vi "main_switch.vi"() -> ()   [LabVIEW 2018]
uses:
  <instrlib>/Keithley 622x LV 2009/Configure/Source/Typedefs/KE622x -- Voltage Limit.ctl
  <instrlib>/Keithley 622x LV 2009/Configure/Output/Typedefs/KE6221 -- Output Response.ctl
  <instrlib>/Keithley 622x LV 2009/Utility/Typedefs/KE622x -- Instrument Type.ctl
  <instrlib>/Keithley 622x LV 2009/Typedefs/KE622x -- On Off Control.ctl
  <instrlib>/Keithley 622x LV 2009/Configure/Source/Typedefs/KE622x -- Current Range.ctl
  <instrlib>/Keithley 622x LV 2009/Configure/Source/Typedefs/KE622x -- Current Ranges.ctl
  <instrlib>/Keithley 622x LV 2009/Configure/Source/Typedefs/KE622x -- Current Level.ctl
  <vilib>/Utility/file.llb/Write Delimited Spreadsheet (string).vi
  <instrlib>/Keithley 622x LV 2009/Keithley 622x.lvlib
  <instrlib>/Keithley 2182/Keithley 2182.lvlib
panel:
  in  "VISA Switch":refnum<visa-resource-name>="GPIB::6"
  out "Close Channel List":string
  in  "Configurations":enum32{"Radio Selection 1", "Radio Selection 2"}(radio)
  out "Iteration number":i32
  out "Current  (A)":dbl
  out "Array Voltage  (V)":dbl
  in  "Voltage Resolution (8)":i32=8
  in  "Range Value (10)":dbl=10.0
  in  "Autorange (T: Enable)":bool=TRUE
  in  "Integration Rate (5)":dbl=5.0
  in  "Integration Rate Units (0: Line Cycles)":i32(ring) items=["Line Cycles", "Seconds"]
  in  "Buffer Count":i32=1
  in  "VISA resource voltage":refnum<visa-resource-name>
  out "Buffer":dbl[](array[numeric])
  out "Buffer Metadata":T1(array[cluster])
  in  "Measurement (0: Voltage Channel 1)":i32(ring) items=["Voltage Channel 1", "Voltage Channel 2"]
  in  "milliseconds to wait":u32=1000
  in  "Step Size":T2=0.001 min=-0.105 max=0.105 format="%.4p"
  in  "End":T2=0.001 min=-0.105 max=0.105 format="%.4p"
  in  "Start":T2=0.001 min=-0.105 max=0.105 format="%.4p"
  in  "Turn Off Output If Voltage Limit?":bool=TRUE
  out "Interlock Tripped?":bool
  out "Voltage Limit?":bool
  in  "Check For SCPI Errors? (T)":bool=TRUE
  in  "Current Range In":T3={"Auto Range?"=TRUE, "Man / Selected\nRange"=enum."2nA"}
  in  "Analog Filter State":T5
  in  "Output Response":T6=enum."Slow"
  in  "Voltage Limit (V)":T7=10.0 min=0.1 max=105.0 step=0.01 format="%.2p"
  out "error at Current off":errorcluster
  out "error at current On":errorcluster
  in  "VISA resource dc ac current source (16)":refnum<visa-resource-name>
  out "Configuration Error":errorcluster
  in  "array":dbl[](array[numeric])
  out "output array":dbl[](array[numeric])
  in  "Instrument Type 2":T8=enum."KE6221"
  # "( select : GPIB0::16::INSTR )"
  # "( select : GPIB0::25::INSTR )"
  # "( select : USB0::0x05E6::0x3706::04368238::INSTR )"
  # "Do Not Enter Buffer Size less than 2"
types:
  T1 = cluster{"Units":string, "Channel":i32, "Channel Type":string}[]
  T2 = typedef "Keithley 622x.lvlib/KE622x -- Current Level.ctl" = dbl
  T3 = typedef "Keithley 622x.lvlib/KE622x -- Current Range.ctl" = cluster{"Auto Range?":bool, "Man / Selected\nRange":T4}
  T4 = typedef "Keithley 622x.lvlib/KE622x -- Current Ranges.ctl" = enum16{"2nA", "20nA", "200nA", "2uA", "20uA", "200uA", "2mA", "20mA", "100mA"}
  T5 = typedef "Keithley 622x.lvlib/KE622x -- On Off Control.ctl" = enum16{"Off", "On"}
  T6 = typedef "Keithley 622x.lvlib/KE6221 -- Output Response.ctl" = enum16{"Fast", "Slow"}
  T7 = typedef "Keithley 622x.lvlib/KE622x -- Voltage Limit.ctl" = dbl
  T8 = typedef "Keithley 622x.lvlib/KE622x -- Instrument Type.ctl" = enum16{"KE6220", "KE6221"}
  T9 = enum16{"Close", "Close Exclusive", "Close Slot Exclusive", "Open", "Open All"}
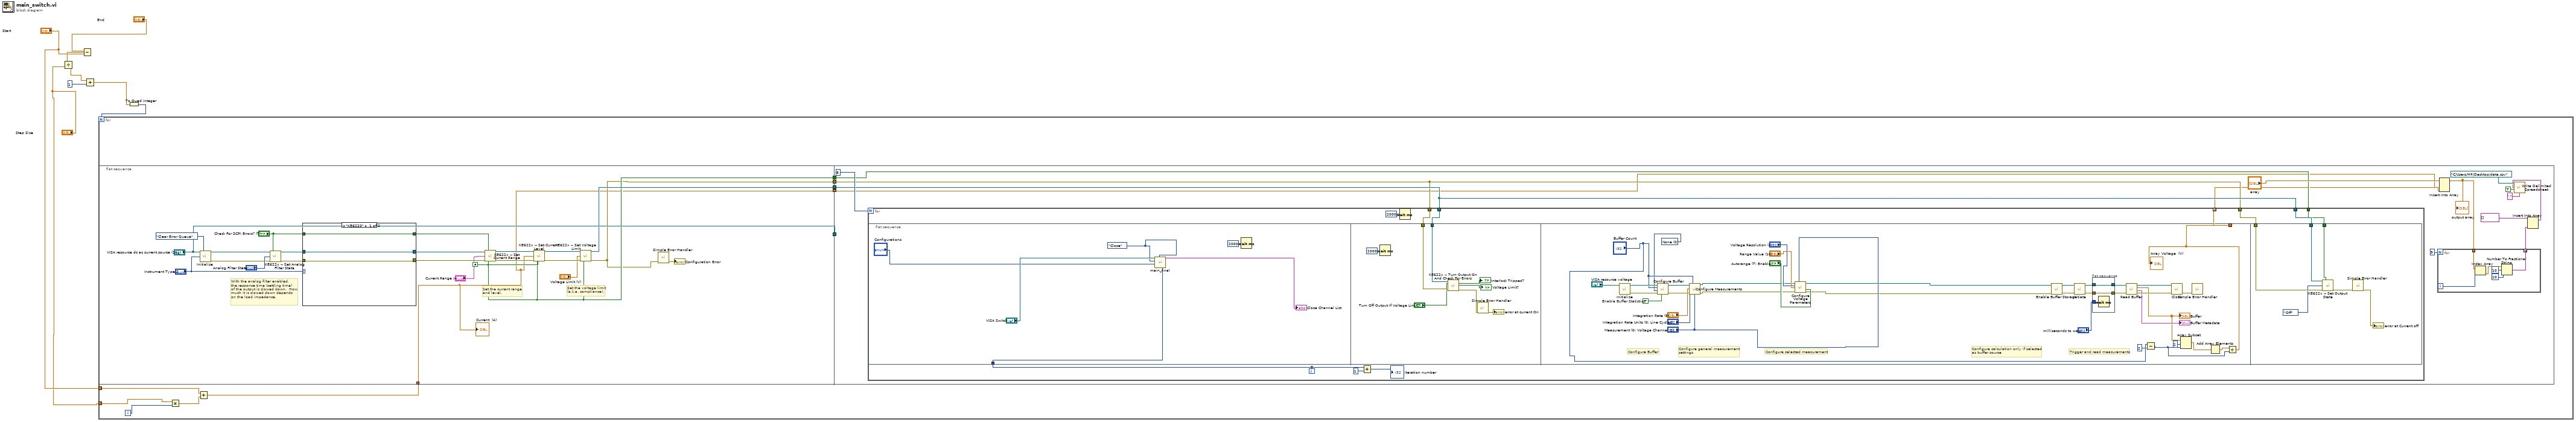
[diagram p0: block diagram]
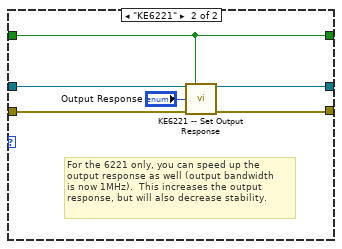
[diagram p2: hidden frame]
diagram:
  n1 = Subtract(x="End", y="Start") -> (x-y=w8:T2)
  n2 = Divide(x=w8, y="Step Size") -> (x/y=w4:T2)
  n3 = Add(x=w4, y=1) -> (x+y=w2:T2)
  n4 = To Quad Integer(1:w2) -> (0:w1:i64)
  n5 = for {
    N: w1 -> [_]
    tunnel: "Step Size" -> [w13]
    tunnel: "Start" -> [w12]
    i -> [w9]
    n6 = flat-sequence {
      tunnel: ["VISA resource dc ac current source (16)"] -> w18
      tunnel: [w22] -> w17
      tunnel: [w20] -> w16
      tunnel: [w21] -> w15
      tunnel: [w19] -> w14
      tunnel: w11 -> [w19]
      tunnel: w18 -> [_]
      tunnel: w17 -> [w63]
      tunnel: w16 -> [w62]
      tunnel: w15 -> [w61]
      tunnel: w14 -> [w51]
      frame #0 {
        w29 = FALSE ("Read Back Set Values? (T)")
        # "Set the voltage limit\n(a.k.a. compliance)."
        # "Set the current range\nand level."
        # "With the analog filter enabled,\nthe response time (settling time)\nof the output is slowed down.  How\nmuch it is slowed down depends\non the load impedance."
        n7 = call <instrlib>:"Initialize.vi"("VISA resource name"="VISA resource dc ac current source (16)", "Error Queue Option"=enum16{"Clear Error Queue", "Error Query"}."Clear Error Queue", "Instrument Type"="Instrument Type 2") -> ("VISA resource name out"=w39:refnum<visa-resource-name>, "error out"=w38:errorcluster)  [unwired: 11 in]
        n8 = call <instrlib>:"KE622x -- Set Analog Filter State.vi"("Resource In"=w39, "Check For SCPI Errors? (T)"="Check For SCPI Errors? (T)", "Analog Filter State"="Analog Filter State", "error in (no error)"=w38) -> ("Resource Out (dupl)"=w37:refnum<visa-resource-name>, "error out"=w35:errorcluster)  [unwired: 10 in]
        n9 = case shown="\"KE6220\"" "Instrument Type 2" {
          tunnel: w37 -> [w43 w50]
          tunnel: w35 -> [w42 w48]
          tunnel: [w43 w47] -> w32
          tunnel: "Check For SCPI Errors? (T)" -> [w44 w46]
          tunnel: [w44 w46] -> w21
          tunnel: [w42 w45] -> w33
          frame "KE6220" {
          }
          frame "KE6221" {
            # "For the 6221 only, you can speed up the\noutput response as well (output bandwidth\nis now 1MHz).  This increases the output\nresponse, but will also decrease stability."
            n10 = call <instrlib>:"KE6221 -- Set Output Response.vi"("Resource In"=w50, "Check For SCPI Errors? (T)"=w46, "KE6221 Output Response"="Output Response", "error in (no error)"=w48) -> ("Resource Out (dupl)"=w47:refnum<visa-resource-name>, "error out"=w45:errorcluster)  [unwired: 10 in]
          }
        }
        n11 = call <instrlib>:"KE622x -- Set Current Range.vi"("Resource In"=w32, "Check For SCPI Errors? (T)"=w21, "Current Range In"="Current Range In", "error in (no error)"=w33, "Read Back Set Values? (T)"=w29) -> ("Resource Out (dupl)"=w31:refnum<visa-resource-name>, "error out"=w30:errorcluster)  [unwired: 8 in, 1 out]
        n12 = call <instrlib>:"KE622x -- Set Current Level.vi"("Resource In"=w31, "Check For SCPI Errors? (T)"=w21, "Current Level (A) In"=w19, "error in (no error)"=w30, "Read Back Set Value? (T)"=w29) -> ("Resource Out (dupl)"=w28:refnum<visa-resource-name>, "error out"=w27:errorcluster)  [unwired: 8 in, 1 out]
        n13 = call <instrlib>:"KE622x -- Set Voltage Limit.vi"("Resource In"=w28, "Check For SCPI Errors? (T)"=w21, "Voltage Limit (V)"="Voltage Limit (V)", "error in (no error)"=w27) -> ("Resource Out (dupl)"=w22:refnum<visa-resource-name>, "error out"=w20:errorcluster)  [unwired: 10 in]
        n14 = call <vilib>:"Simple Error Handler.vi"("error in (no error)"=w20) -> ("error out"=→"Configuration Error":errorcluster)  [unwired: 4 in, 4 out]
        "Current  (A)" <- w19
      }
      frame #1 {
        n15 = for {
          N: 8 -> [_]
          tunnel: [w80] -> w52 mode=indexing
          tunnel: w63 -> [w79]
          tunnel: w62 -> [w78]
          tunnel: w63 -> [w77]
          tunnel: w62 -> [w76]
          tunnel: w61 -> [w75]
          i -> [w73]
          n16 = flat-sequence {
            tunnel: w73 -> [w86]
            tunnel: w79 -> [w95]
            tunnel: w78 -> [w94]
            tunnel: [w96] -> w80
            tunnel: w77 -> [w140]
            tunnel: w76 -> [w139]
            tunnel: w75 -> [w135]
            frame #0 {
              w82 = T9."Close" ("Operation 3")
              n17 = call "main_final.vi"("Numeric"=w86, "Operation 2"=w82, "Radio Buttons"="Configurations", "Operation 3"=w82, "VISA Refnum in"="VISA Switch") -> ("Close Channel List 2"=→"Close Channel List":string)  [unwired: 6 in]
              n18 = Wait (ms)(milliseconds to wait=u32 2000) -> ()  [unwired: 1 out]
            }
            frame #1 {
              n19 = Wait (ms)(milliseconds to wait=u32 2000) -> ()  [unwired: 1 out]
              n20 = call <instrlib>:"KE622x -- Turn Output On And Check For Errors.vi"("Resource In"=w95, "Turn Off Output If Compliance?"="Turn Off Output If Voltage Limit?", "error in (no error)"=w94) -> ("Interlock Tripped?"=→"Interlock Tripped?":bool, "Compliance?"=→"Voltage Limit?":bool, "error out"=w89:errorcluster)  [unwired: 9 in, 1 out]
              n21 = call <vilib>:"Simple Error Handler.vi"("error in (no error)"=w89) -> ("error out"=→"error at current On":errorcluster)  [unwired: 4 in, 4 out]
            }
            frame #2 {
              w105 = 0 items=["None", "Measurements", "Math Calculation"] ("Buffer Source (0: None)")
              w114 = TRUE  # Enable Buffer Statistics
              # "Trigger and read measurements"
              # "Configure general measurement\nsettings"
              # "Configure Buffer"
              # "Configure calculation only if selected\nas buffer source"
              # "Configure selected measurement"
              n22 = call <instrlib>:"Initialize.vi"("VISA resource name"="VISA resource voltage") -> ("error out"=w123:errorcluster, "VISA resource name out"=w122:refnum<visa-resource-name>)  [unwired: 9 in]
              n23 = call <instrlib>:"Configure Buffer.vi"("Enable Buffer Statistics (0: Disable)"=w114, "error in (no error)"=w123, "Buffer Source (0: None)"=w105, "Buffer Size (2)"="Buffer Count", "VISA resource name"=w122) -> ("error out"=w125:errorcluster, "VISA resource name out"=w124:refnum<visa-resource-name>)  [unwired: 5 in]
              n24 = call <instrlib>:"Configure Measurements.vi"("VISA resource name"=w124, "Measurement (0: Voltage Channel 1)"="Measurement (0: Voltage Channel 1)", "Integration Rate (5)"="Integration Rate (5)", "Integration Rate Units (0: Line Cycles)"="Integration Rate Units (0: Line Cycles)", "error in (no error)"=w125, "Sample Count (1)"="Buffer Count") -> ("VISA resource name out"=w100:refnum<visa-resource-name>, "error out"=w99:errorcluster)  [unwired: 8 in]
              n25 = call <instrlib>:"Configure Voltage Parameters.vi"("VISA resource name"=w100, "Measurement (1: Voltage Channel 1)"="Measurement (0: Voltage Channel 1)", "Voltage Resolution (8)"="Voltage Resolution (8)", "Range Value (12)"="Range Value (10)", "Autorange (T: Enable)"="Autorange (T: Enable)", "error in (no error)"=w99) -> ("VISA resource name out"=w97:refnum<visa-resource-name>, "error out"=w98:errorcluster)  [unwired: 8 in]
              n26 = call <instrlib>:"Enable Buffer Storage.vi"("error in (no error)"=w98, "VISA resource name"=w97) -> ("error out"=w121:errorcluster, "VISA resource name out"=w120:refnum<visa-resource-name>)  [unwired: 8 in]
              n27 = call <instrlib>:"Initiate.vi"("error in (no error)"=w121, "VISA resource name"=w120) -> ("error out"=w117:errorcluster, "VISA resource name out"=w115:refnum<visa-resource-name>)  [unwired: 8 in]
              n28 = flat-sequence {
                tunnel: "milliseconds to wait" -> [w134]
                tunnel: [w133] -> w118
                tunnel: w117 -> [w133]
                tunnel: [w132] -> w116
                tunnel: w115 -> [w132]
                frame #0 {
                  n29 = Wait (ms)(milliseconds to wait=w134) -> ()  [unwired: 1 out]
                }
              }
              n30 = call <instrlib>:"Read Buffer.vi"("error in (no error)"=w118, "VISA resource name"=w116) -> ("error out"=w130:errorcluster, "Buffer Metadata"=→"Buffer Metadata":T1, "Buffer"=w112:dbl[], "VISA resource name out"=w129:refnum<visa-resource-name>)  [unwired: 6 in]
              "Buffer" <- w112
              n31 = Subtract(x="Buffer Count", y=2) -> (x-y=w106:i32)
              n32 = call <instrlib>:"Close.vi"("error in (no error)"=w130, "VISA resource name"=w129) -> ("error out"=w113:errorcluster)  [unwired: 9 in]
              n33 = Array Subset(array=w112, index=2, length=w106) -> (w110:dbl[])
              n34 = call <vilib>:"Simple Error Handler.vi"("error in (no error)"=w113) -> ()  [unwired: 4 in, 5 out]
              n35 = Add Array Elements(numeric array=w110) -> (sum=w109:dbl)
              n36 = Divide(x=w109, y=w106) -> (x/y=w96:dbl)
              "Array Voltage  (V)" <- w96
            }
            frame #3 {
              n37 = call <instrlib>:"KE622x -- Set Output State.vi"("Resource In"=w140, "Check For SCPI Errors? (T)"=w135, "Output State"=KE622x_--_On_Off_Control."Off", "error in (no error)"=w139) -> ("error out"=w136:errorcluster)  [unwired: 10 in, 1 out]
              n38 = call <vilib>:"Simple Error Handler.vi"("error in (no error)"=w136) -> ("error out"=→"error at Current off":errorcluster)  [unwired: 4 in, 4 out]
            }
          }
          n39 = Add(x=w73, y=1) -> (x+y=→"Iteration number":i32)
          n40 = Wait (ms)(milliseconds to wait=u32 2000) -> ()  [unwired: 1 out]
        }
        n41 = Insert Into Array(array="array", new element #1=w51, new element #2=w52) -> (w57:dbl[])  [unwired: 1 in]
        "output array" <- w57
        n42 = for {
          N: 9 -> [_]
          tunnel: w57 -> [w71]
          tunnel: [w68] -> w56 mode=indexing
          i -> [w70]
          n43 = Index Array(array=w71, index=w70) -> (element=w69:dbl)
          n44 = Number To Fractional String(number=w69, width (-)=i16 10, precision (6)=i16 10) -> (F-format string=w68:string)  [unwired: 1 in]
        }
        n45 = Insert Into Array(array=string[] [], new element=w56) -> (w54:string[])  [unwired: 1 in]
        n46 = call-poly <vilib>:"Write Delimited Spreadsheet.vi"("file path (dialog if empty)"=path "C:/Users/HP/Desktop/data.csv", "1D data"=w54, "append to file? (new file:F)"=TRUE, "delimiter (\\t)"="," ("delimiter (\\t)")) -> ()  [unwired: 10 in, 2 out]
      }
    }
    n47 = Multiply(x=w13, y=w9) -> (x*y=w10:T2)
    n48 = Add(x=w12, y=w10) -> (x+y=w11:T2)
  }
